vi "Load calibration profile data images.vi"(8 "error in (no error)":errorcluster, 10 "Array":string[][](array[string]), 11 "appended path":path) -> (0 "error out":errorcluster, 2 "Image names":string[](array[string]), 3 "Image Array refs":T1[](array[typedef]))   [LabVIEW 2020]
uses:
  <vilib>/vision/Image Controls.llb/IMAQ Image.ctl
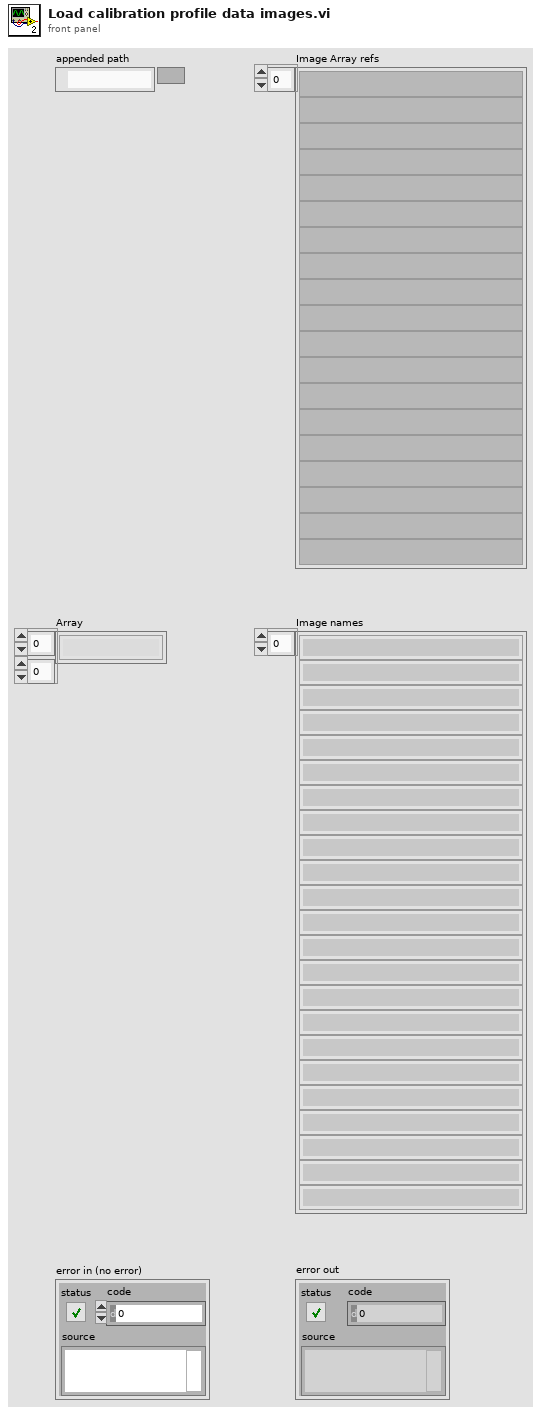
[diagram p1: front panel]
types:
  T1 = typedef "IMAQ Image.ctl" = refnum<image>
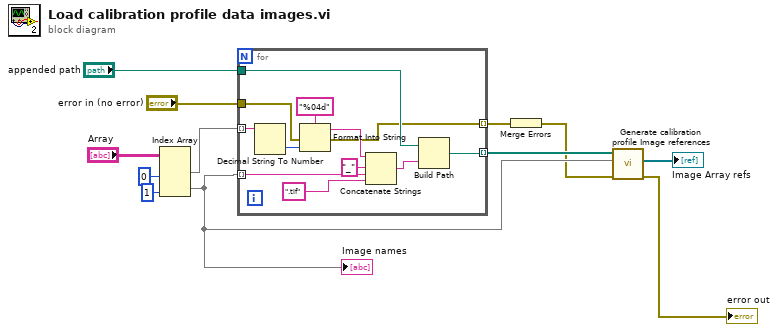
[diagram p0: block diagram]
diagram:
  n1 = Index Array(array="Array", index (col) #1=0 ("disabled index (col)"), index (col) #2=1 ("disabled index (col)")) -> (element #1=w11:string[], element #2=w12:string[])  [unwired: 2 in]
  "Image names" <- w12
  n2 = for {
    tunnel: w12 -> [w24] mode=indexing
    tunnel: "appended path" -> [w21]
    tunnel: [w20] -> w6 mode=indexing
    tunnel: w11 -> [w19] mode=indexing
    tunnel: "error in (no error)" -> [w14]
    tunnel: [w13] -> w2 mode=indexing
    n3 = Decimal String To Number(string=w19) -> (number=w17:i32)  [unwired: 2 in, 1 out]
    n4 = Format Into String(format string="%04d", error in=w14, w17) -> (resulting string=w16:string, error out=w13:errorcluster)  [unwired: 1 in]
    n5 = Concatenate Strings(w16, "_" ("string"), w24, ".tif" ("string")) -> (w22:string)
    n6 = Build Path(base path=w21, name or relative path=w22) -> (appended path=w20:path)
  }
  n7 = Merge Errors(w2) -> (w1:errorcluster)
  n8 = call "Generate calibration profile Image references.vi"("error in (no error)"=w1, "Buffer Image Names"=w12, "File Paths"=w6) -> ("error out"=→"error out":errorcluster, "Image Array refs"=→"Image Array refs":T1[])  [unwired: 7 in]
